vi "Main2.vi"() -> ()   [LabVIEW 2020]
uses:
  Desktop/Servidores LabVIEW/TypeDefs/TypeDEF_MaqEstados.ctl
  <vilib>/Utility/error.llb/DialogType.ctl
  <vilib>/Analysis/5stat.llb/RMS (DBL).vi
  cedfa54c-138c-4538-9d6c-e86a0f259f6c.vi
  Desktop/Servidores LabVIEW/TypeDefs/Global_Parara.vi
  <vilib>/Utility/SystemLogging/NI_SystemLogging.lvlib
  <vilib>/Utility/TDMS File Viewer/NI_TDMS File Viewer.lvlib
  <vilib>/Analysis/NI_AALPro.lvlib
panel:
  out "File Path":path
  out "Messages":string
  out "Waveform Chart - Dark":dbl(graph)
  out "Notification Data Base Loop":bool
  out "Notification Process Loop":bool
  out "Notification SIEMENS PLC Loop":bool
  out "Notification AB PLC Loop":bool
  out "Torque Out":dbl
  in  "Torque In 2":dbl
  in  "Torque In":dbl
  in  "Tabs Buttons":enum32{"Button 1", "Button 2", "Button 3"}(radio) caption="Radio Buttons - Customizable"
  in  "Abort Button":bool
  out "Tab Control":enum32{"Page 1", "Page 2", "Page 3"}(tab)
  in  "Open Square":bool
  in  "Delete Tool":bool
  in  "Start Tool":bool
  in  "Pause Tool":bool
  in  "Save Tool 2":bool
  out "# elements in queue":i32
  out "Waveform Chart - Dark 2":dbl(graph) caption="Waveform Chart - Dark"
  in  "File Path":path
  in  "Path Image Control":path
  in  "Limit Control":dbl min=0.0
  in  "Refresh Button":bool
  out "Table":string[][](table)
  in  "Orden":string(combo)
  in  "Elemento":string(combo)
  out "error out":errorcluster
  # "Debugging Aditional Items"
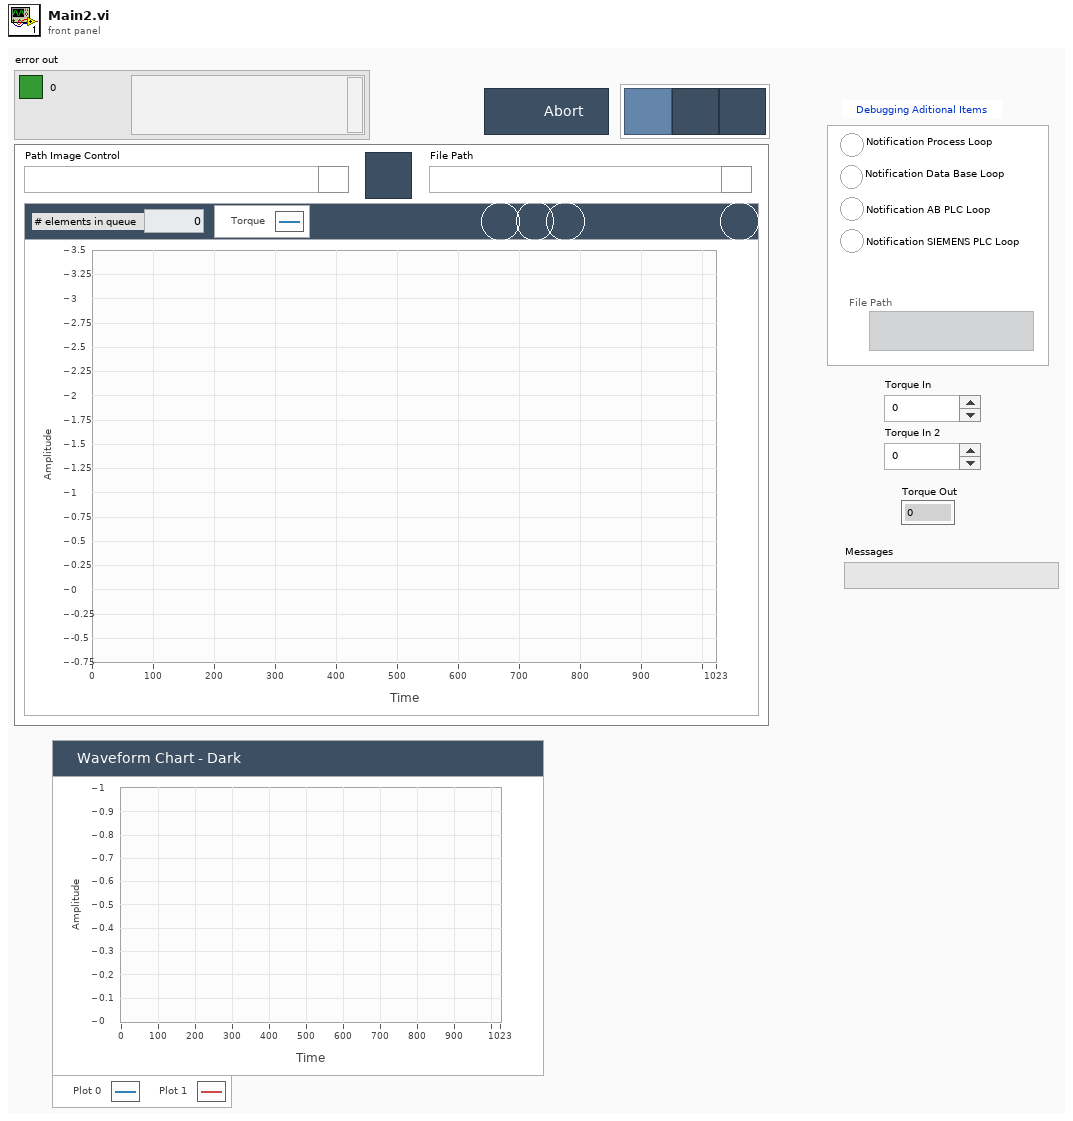
[diagram p1: front panel]
types:
  T1 = typedef "TypeDEF_MaqEstados.ctl" = enum16{"Startfing Up", "Adquisition", "Save", "Fault"}
  T2 = enum8{"Enabled", "Disabled", "Disabled and Grayed Out"}
  T3 = typedef "DialogType.ctl" = u16
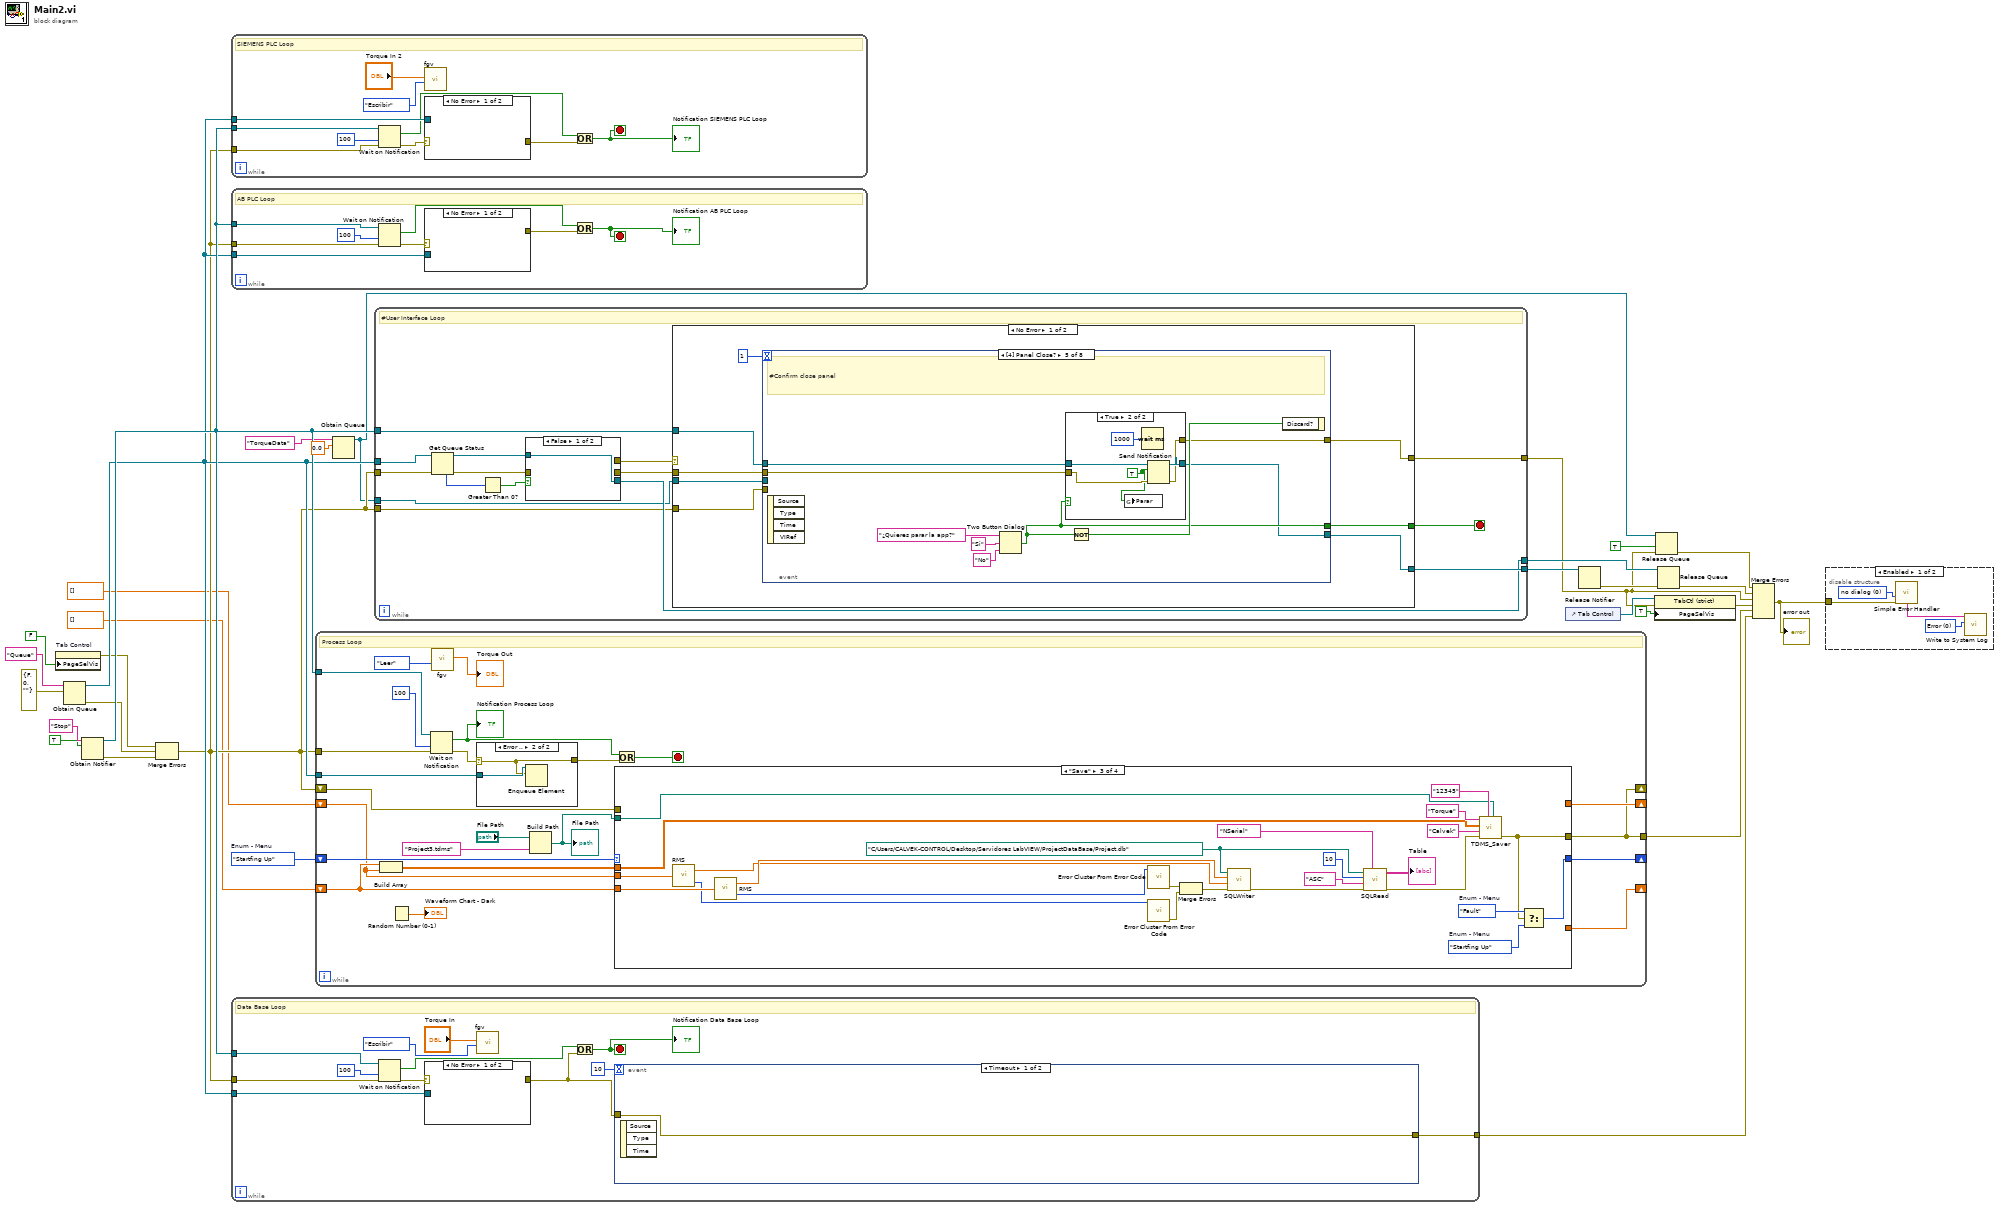
[diagram p0: block diagram]
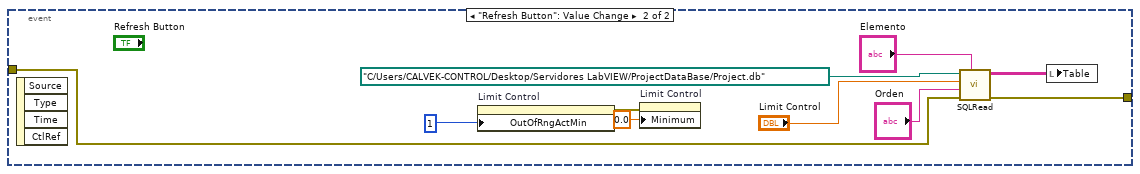
[diagram p3: hidden frame]
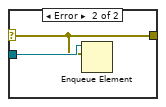
[diagram p4: hidden frame]
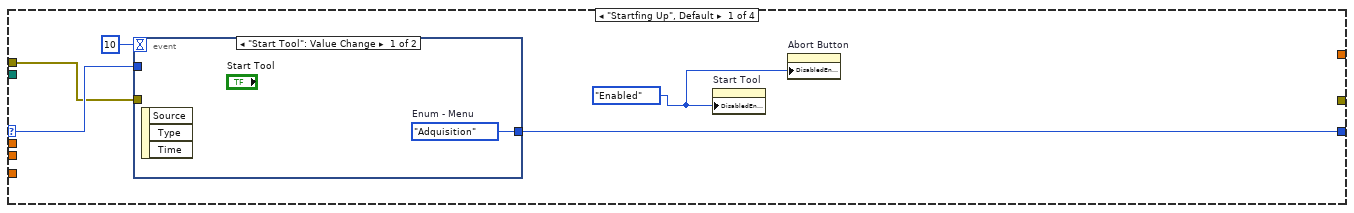
[diagram p5: hidden frame]
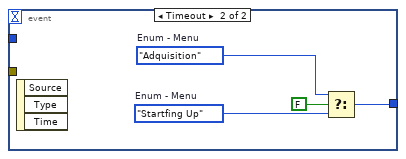
[diagram p6: hidden frame]
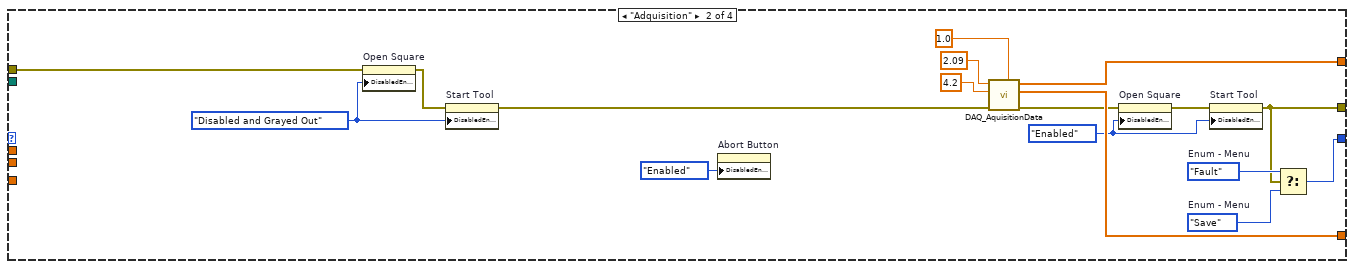
[diagram p7: hidden frame]
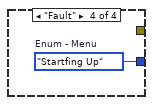
[diagram p8: hidden frame]
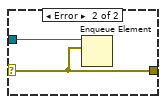
[diagram p10: hidden frame]
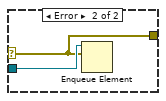
[diagram p11: hidden frame]
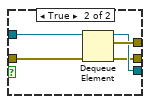
[diagram p12: hidden frame]
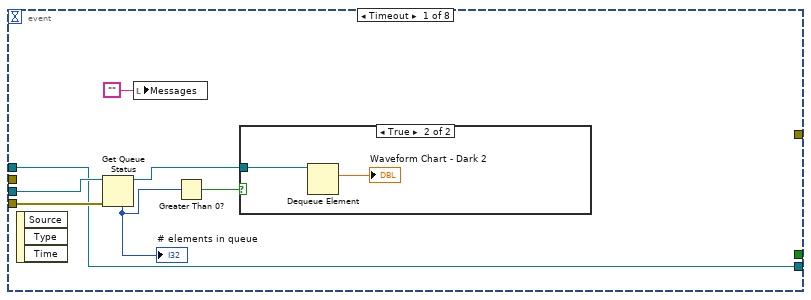
[diagram p13: hidden frame]
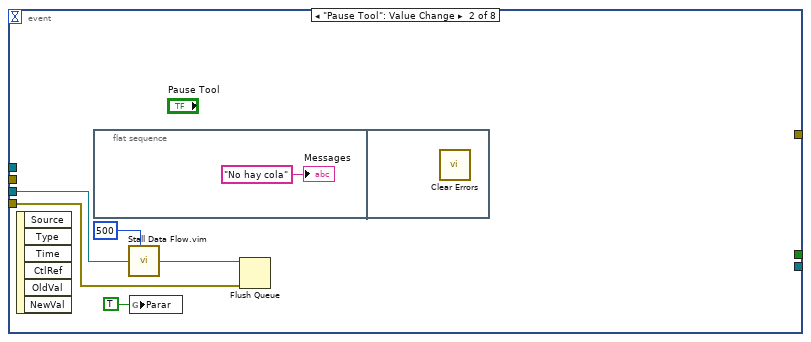
[diagram p15: hidden frame]
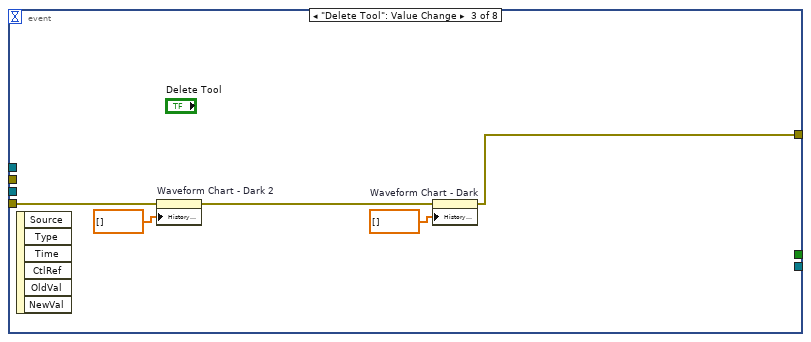
[diagram p16: hidden frame]
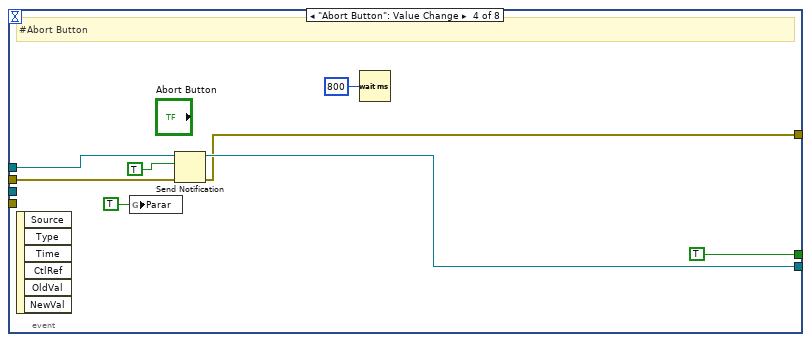
[diagram p17: hidden frame]
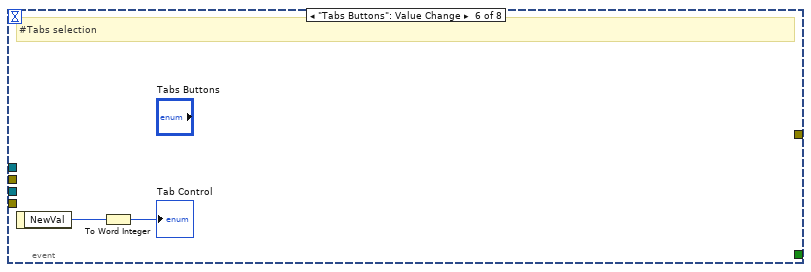
[diagram p19: hidden frame]
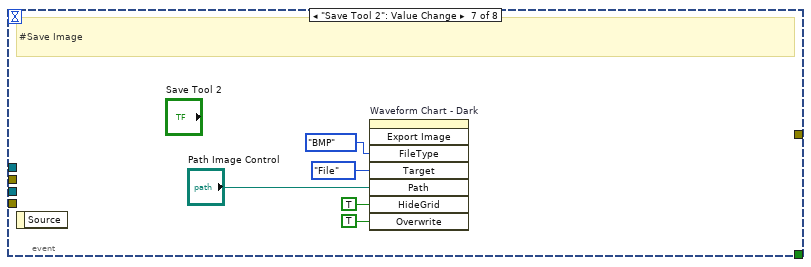
[diagram p20: hidden frame]
diagram:
  w12 = TypeDEF_MaqEstados."Startfing Up"  # Enum - Menu
  n1 = property on="Tab Control" class="TabCtl (strict)"("PageSelVis"=FALSE ("Page Selector Visible")) -> (error out=w19:errorcluster)  [unwired: 2 in, 1 out]
  n2 = Obtain Queue(name (unnamed)="Queue", element data type=errorcluster {"status"=FALSE, "code"=0, "source"=""} ("error constant")) -> (queue out=w24:refnum<queue>, error out=w23:errorcluster)  [unwired: 3 in, 1 out]
  n3 = Obtain Notifier(name (unnamed)="Stop", notification data type=TRUE) -> (notifier out=w27:refnum<notifier>, error out=w22:errorcluster)  [unwired: 2 in, 1 out]
  n4 = Merge Errors(w19, w23, w22) -> (w10:errorcluster)
  n5 = while {
    tunnel: w27 -> [w40]
    tunnel: w24 -> [w37]
    tunnel: w10 -> [w38]
    stop <- w34 stop-if-true
    # "SIEMENS PLC Loop"
    n6 = Wait on Notification(notifier=w40, timeout in ms (-1)=100, error in (no error)=w38) -> (notification=w35:bool, error out=w36:errorcluster)  [unwired: 1 in, 2 out]
    n7 = call "fgv.vi"("Selector FGV"=enum16{"Leer", "Escribir"}."Escribir", "Torque In"="Torque In 2") -> ()  [unwired: 9 in, 1 out]
    n8 = case shown="No Error" w36 {
      selector: w36 -> [_ w41]
      tunnel: w37 -> [_ w42]
      tunnel: [_ w41] -> w33
      frame No Error {
      }
      frame Error {
        n9 = Enqueue Element(queue=w42, element=w41) -> ()  [unwired: 2 in, 3 out]
      }
    }
    n10 = Or(x=w35, y=w33) -> (x .or. y?=w34:bool)
    "Notification SIEMENS PLC Loop" <- w34
  }
  n11 = while {
    tunnel: w27 -> [w50]
    tunnel: w24 -> [w47]
    tunnel: w10 -> [w48]
    stop <- w45 stop-if-true
    # "AB PLC Loop"
    n12 = Wait on Notification(notifier=w50, timeout in ms (-1)=100, error in (no error)=w48) -> (notification=w44:bool, error out=w46:errorcluster)  [unwired: 1 in, 2 out]
    n13 = case shown="No Error" w46 {
      selector: w46 -> [_ w51]
      tunnel: w47 -> [_ w52]
      tunnel: [_ w51] -> w43
      frame No Error {
      }
      frame Error {
        n14 = Enqueue Element(queue=w52, element=w51) -> ()  [unwired: 2 in, 3 out]
      }
    }
    n15 = Or(x=w44, y=w43) -> (x .or. y?=w45:bool)
    "Notification AB PLC Loop" <- w45
  }
  n16 = while {
    tunnel: w27 -> [w64]
    tunnel: w24 -> [w62]
    tunnel: w10 -> [w61]
    tunnel: [w54] -> w1
    stop <- w59 stop-if-true
    # "Data Base Loop"
    n17 = Wait on Notification(notifier=w64, timeout in ms (-1)=100, error in (no error)=w61) -> (notification=w58:bool, error out=w60:errorcluster)  [unwired: 1 in, 2 out]
    n18 = case shown="No Error" w60 {
      selector: w60 -> [_ w76]
      tunnel: w62 -> [_ w77]
      tunnel: [_ w76] -> w55
      frame No Error {
      }
      frame Error {
        n19 = Enqueue Element(queue=w77, element=w76) -> ()  [unwired: 2 in, 3 out]
      }
    }
    n20 = call "fgv.vi"("Selector FGV"=enum16{"Leer", "Escribir"}."Escribir", "Torque In"="Torque In") -> ()  [unwired: 9 in, 1 out]
    n21 = Or(x=w58, y=w55) -> (x .or. y?=w59:bool)
    "Notification Data Base Loop" <- w59
    n22 = event shown="[0] Timeout" {
      selector: _ -> [_ _]
      dyn-events: _ -> [_ _]
      timeout: 10 -> [_ _]
      tunnel: w55 -> [w65 w73]
      tunnel: [w65 w72] -> w54
      event Timeout {
        n23 = event-data() -> ()  [unwired: 1 in, 3 out]
      }
      event "Refresh Button": Value Change {
        n24 = event-data() -> ()  [unwired: 1 in, 4 out]
        n25 = property on="Limit Control" class="DigNum (strict)"("OutOfRngActMin"=u8 1 ("Response to Value Outside Limits:Maximum")) -> (error out=w67:errorcluster)  [unwired: 2 in, 1 out]
        n26 = property on="Limit Control" class="DigNum (strict)"(error in=w67, "Minimum"=0.0 ("Data Entry Limits:Minimum")) -> ()  [unwired: 1 in, 2 out]
        n27 = call "SQLRead.vi"("Elemento"="Elemento", "error in (no error)"=w73, "Orden"="Orden", "Numero de elementos"="Limit Control", "Path Control"=path "C:/Users/CALVEK-CONTROL/Desktop/Servidores LabVIEW/ProjectDataBase/Project.db") -> ("error out"=w72:errorcluster, "Table"=w69:string[][])  [unwired: 5 in]
        n28 = local write "Table"(w69) -> ()
      }
    }
  }
  n29 = while {
    tunnel: w27 -> [w100]
    tunnel: w24 -> [w97]
    tunnel: w10 -> [w98]
    shift-right: [w90] -> _
    shift-left: w12 -> [w91]
    tunnel: [w80] -> w9
    shift-right: [w86] -> _
    shift-left: dbl[] [] ("ForceArray") -> [w78]
    shift-right: [w85] -> _
    shift-left: dbl[] [] ("TorqueArray") -> [w79]
    shift-right: [w80] -> _
    shift-left: w10 -> [w87]
    stop <- w95 stop-if-true
    # "Process Loop"
    n30 = Build Array(w79, w78) -> (w84:dbl[][])
    n31 = Random Number (0-1)() -> (number: 0 to 1=→"Waveform Chart - Dark":dbl)
    n32 = Wait on Notification(notifier=w100, timeout in ms (-1)=100, error in (no error)=w98) -> (notification=w94:bool, error out=w92:errorcluster)  [unwired: 1 in, 2 out]
    "Notification Process Loop" <- w94
    n33 = call "fgv.vi"("Selector FGV"=enum16{"Leer", "Escribir"}."Leer") -> ("Torque Out"=→"Torque Out":dbl)  [unwired: 10 in]
    n34 = case shown="Error .." w92 {
      selector: w92 -> [_ w154]
      tunnel: w97 -> [_ w155]
      tunnel: [_ w154] -> w96
      frame No Error {
      }
      frame Error {
        n35 = Enqueue Element(queue=w155, element=w154) -> ()  [unwired: 2 in, 3 out]
      }
    }
    n36 = Build Path(base path="File Path", name or relative path="Project3.tdms" ("Title")) -> (appended path=w83:path)
    "File Path" <- w83
    n37 = case shown="\"Save\"" w91 {
      selector: w91 -> [w105 _ _ _]
      tunnel: [w104 w125 w150 w153] -> w90
      tunnel: w87 -> [w103 w117 _ _]
      tunnel: [_ w123 w135 _] -> w80
      tunnel: [_ w120 _ _] -> w86
      tunnel: [_ w119 _ _] -> w85
      tunnel: w84 -> [_ _ w148 _]
      tunnel: w83 -> [_ _ w145 _]
      tunnel: w79 -> [_ _ w144 _]
      tunnel: w78 -> [_ _ w141 _]
      frame "Startfing Up", Default {
        w101 = T2."Enabled" ("Disabled")
        n38 = event shown="[0] \"Start Tool\": Value Change" {
          selector: _ -> [_ _]
          dyn-events: _ -> [_ _]
          timeout: 10 -> [_ _]
          tunnel: w105 -> [_ _]
          tunnel: [w106 w108] -> w104
          tunnel: w103 -> [_ _]
          event "Start Tool": Value Change {
            w106 = TypeDEF_MaqEstados."Adquisition"  # Enum - Menu
            n39 = event-data() -> ()  [unwired: 1 in, 3 out]
          }
          event Timeout {
            w109 = TypeDEF_MaqEstados."Startfing Up"  # Enum - Menu
            w110 = TypeDEF_MaqEstados."Adquisition"  # Enum - Menu
            n40 = event-data() -> ()  [unwired: 1 in, 3 out]
            n41 = Select(t=w110, s=FALSE, f=w109) -> (s? t:f=w108:T1)
          }
        }
        n42 = property on="Start Tool" class="Bool"("DisabledEnum"=w101) -> ()  [unwired: 2 in, 2 out]
        n43 = property on="Abort Button" class="Bool"("DisabledEnum"=w101) -> ()  [unwired: 2 in, 2 out]
      }
      frame "Adquisition" {
        w112 = T2."Enabled" ("Disabled")
        w115 = T2."Disabled and Grayed Out" ("Disabled")
        w126 = TypeDEF_MaqEstados."Save"  # Enum - Menu
        w127 = TypeDEF_MaqEstados."Fault"  # Enum - Menu
        n44 = property on="Open Square" class="Bool"(error in=w117, "DisabledEnum"=w115) -> (error out=w116:errorcluster)  [unwired: 1 in, 1 out]
        n45 = property on="Start Tool" class="Bool"(error in=w116, "DisabledEnum"=w115) -> (error out=w124:errorcluster)  [unwired: 1 in, 1 out]
        n46 = property on="Abort Button" class="Bool"("DisabledEnum"=T2."Enabled" ("Disabled")) -> ()  [unwired: 2 in, 2 out]
        n47 = call "DAQ_AquisitionData.vi"("Numeric Control"=1.0, "error in (no error)"=w124, "b"=4.2, "m"=2.09) -> ("error IO"=w114:errorcluster, "TorqueArray"=w119:dbl[], "ForceArray"=w120:dbl[])  [unwired: 5 in]
        n48 = property on="Open Square" class="Bool"(error in=w114, "DisabledEnum"=w112) -> (error out=w113:errorcluster)  [unwired: 1 in, 1 out]
        n49 = property on="Start Tool" class="Bool"(error in=w113, "DisabledEnum"=w112) -> (error out=w123:errorcluster)  [unwired: 1 in, 1 out]
        n50 = Select(t=w127, s=w123, f=w126) -> (s? t:f=w125:T1)
      }
      frame "Save" {
        w132 = path "C:/Users/CALVEK-CONTROL/Desktop/Servidores LabVIEW/ProjectDataBase/Project.db" ("Path Control")
        w152 = TypeDEF_MaqEstados."Startfing Up"  # Enum - Menu
        w151 = TypeDEF_MaqEstados."Fault"  # Enum - Menu
        n51 = call-poly <vilib>:"RMS.vi"("X"=w141) -> ("rms value"=w136:dbl, "error"=w137:i32)
        n52 = call-poly <vilib>:"RMS.vi"("X"=w144) -> ("rms value"=w143:dbl, "error"=w142:i32)
        n53 = call <vilib>:"Error Cluster From Error Code.vi"("error code (0)"=w142) -> ("error out"=w140:errorcluster)  [unwired: 8 in]
        n54 = call <vilib>:"Error Cluster From Error Code.vi"("error code (0)"=w137) -> ("error out"=w139:errorcluster)  [unwired: 8 in]
        n55 = Merge Errors(w140, w139) -> (w138:errorcluster)
        n56 = call "SQLWriter.vi"("error in (no error)"=w138, "Force RMS"=w136, "Torque RMS"=w143, "Path Control"=w132) -> ("error out"=w134:errorcluster)  [unwired: 7 in]
        n57 = call "SQLRead.vi"("Elemento"="NSerial", "error in (no error)"=w134, "Orden"="ASC", "Numero de elementos"=10, "Path Control"=w132) -> ("error out"=w133:errorcluster, "Table"=→"Table":string[][])  [unwired: 5 in]
        n58 = call "TDMS_Saver.vi"("Path Control"=w145, "Serial Number"="12345", "error in (no error)"=w133, "Author"="Calvek", "2D Array"=w148, "Title"="Torque") -> ("error out"=w135:errorcluster)  [unwired: 5 in]
        n59 = Select(t=w151, s=w135, f=w152) -> (s? t:f=w150:T1)
      }
      frame "Fault" {
        w153 = TypeDEF_MaqEstados."Startfing Up"  # Enum - Menu
      }
    }
    n60 = Or(x=w94, y=w96) -> (x .or. y?=w95:bool)
  }
  n61 = Obtain Queue(name (unnamed)="TorqueData", element data type=0.0) -> (queue out=w4:refnum<queue>)  [unwired: 3 in, 2 out]
  n62 = while {
    tunnel: w27 -> [w169]
    tunnel: [w168] -> w28
    tunnel: w24 -> [w164]
    tunnel: w10 -> [w158]
    tunnel: [w163] -> w6
    tunnel: [w161] -> w14
    tunnel: w4 -> [w160]
    tunnel: w10 -> [w159]
    stop <- w170 stop-if-true
    # "#User Interface Loop"
    n63 = Get Queue Status(queue=w164, error in (no error)=w158) -> (queue out=w162:refnum<queue>, error out=w157:errorcluster, # elements in queue=w166:i32)  [unwired: 1 in, 5 out]
    n64 = Greater Than 0?(x=w166) -> (x > 0?=w165:bool)
    n65 = case shown="False" w165 {
      tunnel: [_ w176] -> w167
      tunnel: w162 -> [w171 w175]
      tunnel: [w171 w174] -> w161
      tunnel: w157 -> [_ w173]
      tunnel: [_ w172] -> w156
      frame False {
      }
      frame True {
        n66 = Dequeue Element(queue=w175, error in (no error)=w173) -> (queue out=w174:refnum<queue>, element=w176:errorcluster, error out=w172:errorcluster)  [unwired: 1 in, 1 out]
      }
    }
    n67 = case shown="No Error" w167 {
      selector: w167 -> [_ w240]
      tunnel: [w184 TRUE ("T button?")] -> w170
      tunnel: w169 -> [w183 w246]
      tunnel: [w182 w243] -> w168
      tunnel: w156 -> [w180 _]
      tunnel: [w179 w241] -> w163
      tunnel: w160 -> [w178 _]
      tunnel: w159 -> [w177 _]
      frame No Error {
        n68 = event shown="[4] Panel Close?" {
          selector: _ -> [_ _ _ _ _ _ _ _]
          dyn-events: _ -> [_ _ _ _ _ _ _ _]
          timeout: 1 -> [_ _ _ _ _ _ _ _]
          tunnel: [_ _ _ TRUE ("Abort Button") w217 _ _ _] -> w184
          tunnel: w183 -> [w186 _ _ w210 w216 _ _ _]
          tunnel: [w186 _ _ w209 w215 _ _ _] -> w182
          tunnel: w180 -> [_ _ _ w208 w214 _ _ w238]
          tunnel: [_ _ w201 w207 w213 _ _ w237] -> w179
          tunnel: w178 -> [w191 w196 _ _ _ _ _ _]
          tunnel: w177 -> [w190 w197 w204 _ _ _ _ _]
          event Timeout {
            n69 = event-data() -> ()  [unwired: 1 in, 3 out]
            n70 = Get Queue Status(queue=w191, error in (no error)=w190) -> (queue out=w189:refnum<queue>, # elements in queue=w188:i32)  [unwired: 1 in, 6 out]
            "# elements in queue" <- w188
            n71 = local write "Messages"("") -> ()
            n72 = Greater Than 0?(x=w188) -> (x > 0?=w187:bool)
            n73 = case shown="True" w187 {
              tunnel: w189 -> [_ w192]
              frame False {
              }
              frame True {
                n74 = Dequeue Element(queue=w192) -> (element=→"Waveform Chart - Dark 2":dbl)  [unwired: 2 in, 3 out]
              }
            }
          }
          event "Pause Tool": Value Change {
            n75 = event-data() -> ()  [unwired: 1 in, 6 out]
            n76 = flat-sequence {
              frame #0 {
                "Messages" <- "No hay cola" ("String Control")
              }
              frame #1 {
                n77 = call <vilib>:"Clear Errors.vi"() -> ()  [unwired: 6 in, 2 out]
              }
            }
            n78 = call "Stall Data Flow.vim"("value in"=w196, "milliseconds to wait"=u32 500) -> ("value out"=w195:refnum<queue>)  [unwired: 1 out]
            n79 = global write "Global_Parara.vi" "Parar"(TRUE ("Parar")) -> ()
            n80 = Flush Queue(queue=w195, error in (no error)=w197) -> ()  [unwired: 3 out]
          }
          event "Delete Tool": Value Change {
            n81 = event-data() -> ()  [unwired: 1 in, 6 out]
            n82 = property on="Waveform Chart - Dark 2" class="WFChart (strict)"(error in=w204, "History Data"=dbl[] []) -> (error out=w202:errorcluster)  [unwired: 1 in, 1 out]
            n83 = property on="Waveform Chart - Dark" class="WFChart (strict)"(error in=w202, "History Data"=dbl[] []) -> (error out=w201:errorcluster)  [unwired: 1 in, 1 out]
          }
          event "Abort Button": Value Change {
            # "#Abort Button"
            n84 = event-data() -> ()  [unwired: 1 in, 6 out]
            n85 = global write "Global_Parara.vi" "Parar"(TRUE ("Parar")) -> ()
            n86 = Send Notification(notification=TRUE, notifier=w210, error in (no error)=w208) -> (notifier out=w209:refnum<notifier>, error out=w207:errorcluster)
            n87 = Wait (ms)(milliseconds to wait=u32 800) -> ()  [unwired: 1 out]
          }
          event Panel Close? {
            # "#Confirm close panel"
            n88 = event-data() -> ()  [unwired: 1 in, 4 out]
            n89 = Two Button Dialog(message="¿Quieres parar la app?", 1:"No" ("F button name (\"Cancel\")"), 2:"Si" ("T button name (\"OK\")")) -> (T button?=w217:bool)
            n90 = case shown="True" w217 {
              tunnel: w216 -> [w222 w228]
              tunnel: [w222 w227] -> w215
              tunnel: w214 -> [_ w225]
              tunnel: [_ w224] -> w213
              frame False {
              }
              frame True {
                w223 = TRUE
                n91 = global write "Global_Parara.vi" "Parar"(w223) -> ()
                n92 = Wait (ms)(milliseconds to wait=u32 1000) -> ()  [unwired: 1 out]
                n93 = Send Notification(notification=w223, notifier=w228, error in (no error)=w225) -> (notifier out=w227:refnum<notifier>, error out=w224:errorcluster)
              }
            }
            n94 = Not(x=w217) -> (.not. x?=w218:bool)
            n95 = event-data("Discard?"=w218) -> ()  [unwired: 1 in, 1 out]
          }
          event "Tabs Buttons": Value Change {
            # "#Tabs selection"
            n96 = event-data() -> ("NewVal"=w229:enum32{"Button 1", "Button 2", "Button 3"})  [unwired: 1 in]
            n97 = To Word Integer(number=w229) -> (16bit integer=→"Tab Control":i16)
          }
          event "Save Tool 2": Value Change {
            # "#Save Image"
            n98 = event-data() -> ()  [unwired: 1 in, 1 out]
            n99 = invoke on="Waveform Chart - Dark" class="WFChart (strict)" method="Export Image"("FileType"=enum32{"BMP", "EPS", "EMF", "PICT"}."BMP" ("File Type"), "Target"=enum32{"File", "Clipboard"}."File", "Path"="Path Image Control", "HideGrid"=TRUE ("Hide Grid"), "Overwrite"=TRUE ("Always Overwrite")) -> ()  [unwired: 3 in, 8 out]
          }
          event "Open Square": Value Change {
            n100 = event-data() -> ()  [unwired: 1 in, 3 out]
            n101 = local read "File Path"() -> (w236:path)
            n102 = call <vilib>:"TDMS - File Viewer (NXG Style).vi"("error in"=w238, "file in"=w236) -> ("error out"=w237:errorcluster)  [unwired: 8 in, 1 out]
          }
        }
      }
      frame Error {
        n103 = Send Notification(notification=TRUE, notifier=w246) -> (notifier out=w243:refnum<notifier>, error out=w242:errorcluster)  [unwired: 1 in]
        n104 = Wait (ms)(milliseconds to wait=u32 800) -> ()  [unwired: 1 out]
        n105 = Merge Errors(w242, w240) -> (w241:errorcluster)
      }
    }
  }
  n106 = control-ref of="Tab Control"() -> (w13:refnum<vi>)
  n107 = Release Notifier(notifier=w28) -> (error out=w16:errorcluster)  [unwired: 2 in, 2 out]
  n108 = property on="Property Node" class="TabCtl (strict)"(reference=w13, error in=w6, "PageSelVis"=TRUE ("Page Selector Visible")) -> (error out=w17:errorcluster)  [unwired: 1 out]
  n109 = Release Queue(queue=w4, force destroy? (F)=TRUE, error in (no error)=w6) -> (error out=w5:errorcluster)  [unwired: 2 out]
  n110 = Release Queue(queue=w14, error in (no error)=w16) -> (error out=w15:errorcluster)  [unwired: 1 in, 2 out]
  n111 = Merge Errors(w5, w15, w6, w17, w9, w1) -> (w21:errorcluster)
  "error out" <- w21
  n112 = disable-structure shown="Enabled" {
    disable-tunnel: w21 -> [w247 _]
    frame Enabled {
      w249 = 0 items=["Error", "Warning", "Informational"] ("severity")
      w250 = T3 0 items=["no dialog", "OK message", "continue or stop message", "OK message + warnings", "continue/stop + warnings"] ("type of dialog (OK msg:1)")
      n113 = call <vilib>:"Simple Error Handler.vi"("type of dialog (OK msg:1)"=w250, "error in (no error)"=w247) -> ("message"=w248:string)  [unwired: 3 in, 4 out]
      n114 = call <vilib>:"Write to System Log.vi"("severity"=w249, "message"=w248) -> ()  [unwired: 9 in, 1 out]
    }
    frame Disabled {
    }
  }
